vi "Get Magnet Vector Field.vi"(8 "error in (no error)":errorcluster, 11 "Instrument.VRM in":refnum<class "Instrument.OxfordVRM.lvclass">) -> (0 "error out":errorcluster, 1 "status":string, 2 "Magnet Field (T)":dbl[](array[numeric]), 3 "Instrument.VRM out":refnum<class "Instrument.OxfordVRM.lvclass">, 4 "finished":bool)   [LabVIEW 2019, in "Instrument.OxfordVRM.lvclass"]
uses:
  Instrument.OxfordVRM.lvclass
  Typedefs/Instrument.VRM.publicCommands-enum.ctl
  Typedefs/VRM Magnet Axis--Enum.ctl
  5e873d59-b7fa-4b76-b36a-7150f831c1b5.vi
  Typedefs/Instrument.VRM.getMagnetVector-cluster.ctl
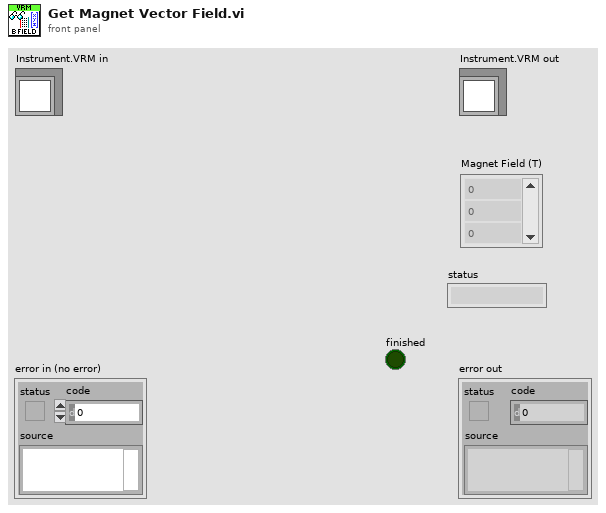
[diagram p1: front panel]
types:
  T1 = typedef "Instrument.OxfordVRM.lvclass/Instrument.VRM.getMagnetVector-cluster.ctl" = cluster{"field":dbl[], "status":string, "finished":bool}
  T2 = typedef "Instrument.OxfordVRM.lvclass/VRM Magnet Axis--Enum.ctl" = enum16{"Z", "X", "Y", "ALL"}
  T3 = typedef "Instrument.OxfordVRM.lvclass/Instrument.VRM.publicCommands-enum.ctl" = enum16{"setMagnet", "setMagnetVector", "getMagnet", "getMagnetVector"}
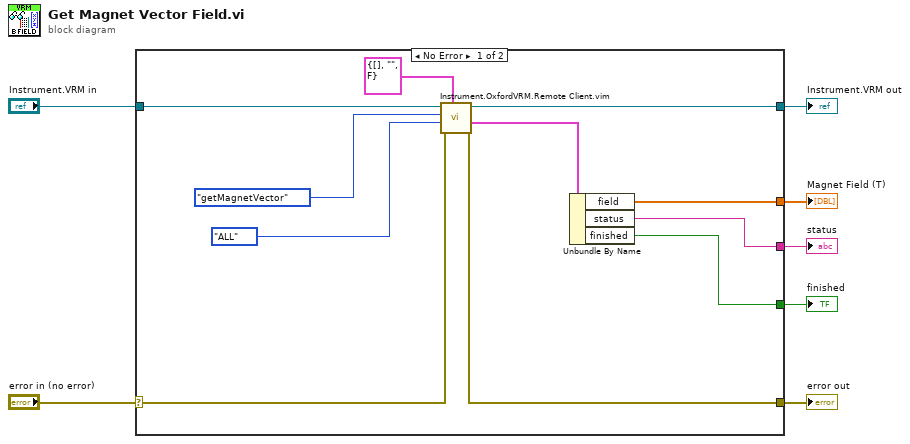
[diagram p0: block diagram]
diagram:
  n1 = case shown="No Error" "error in (no error)" {
    selector: "error in (no error)" -> [w16 w20]
    tunnel: [w14 w20] -> w7
    tunnel: "Instrument.VRM in" -> [w18 w19]
    tunnel: [w17 w19] -> w5
    tunnel: [w10 _] -> w3
    tunnel: [w9 _] -> w2
    tunnel: [w8 _] -> w1
    frame No Error {
      n2 = call "Instrument.OxfordVRM.Remote Client.vim"("Data Out type"=T1 {"field"=[], "status"="", "finished"=FALSE} ("getMagnetVector"), "error in (no error)"=w16, "Data"=VRM_Magnet_Axis--Enum."ALL" ("Axis"), "Commands"=Instrument.VRM.publicCommands-enum."getMagnetVector", "Instrument.VRM in"=w18) -> ("error out"=w14:errorcluster, "Data out"=w11:T1, "Instrument.VRM out"=w17:refnum<class "Instrument.OxfordVRM.lvclass">)  [unwired: 4 in]
      n3 = Unbundle By Name(w11) -> ("field"=w10:dbl[], "status"=w9:string, "finished"=w8:bool)
    }
    frame Error {
    }
  }
  "Instrument.VRM out" <- w5
  "Magnet Field (T)" <- w3
  "error out" <- w7
  "status" <- w2
  "finished" <- w1
